vi "MGCC_StaEst_main.vi"() -> ()   [LabVIEW 2016]
panel:
  out "Boolean 7":bool
  out "Boolean 6":bool
  out "Boolean 5":bool
  out "Boolean 4":bool
  out "Boolean 3":bool
  out "Boolean 2":bool
  out "Boolean":bool
  out "Boolean":bool
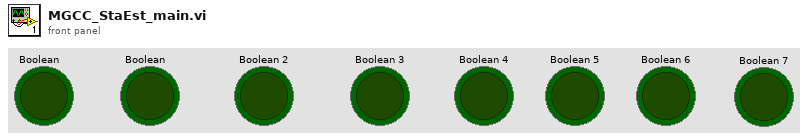
[diagram p1: front panel]
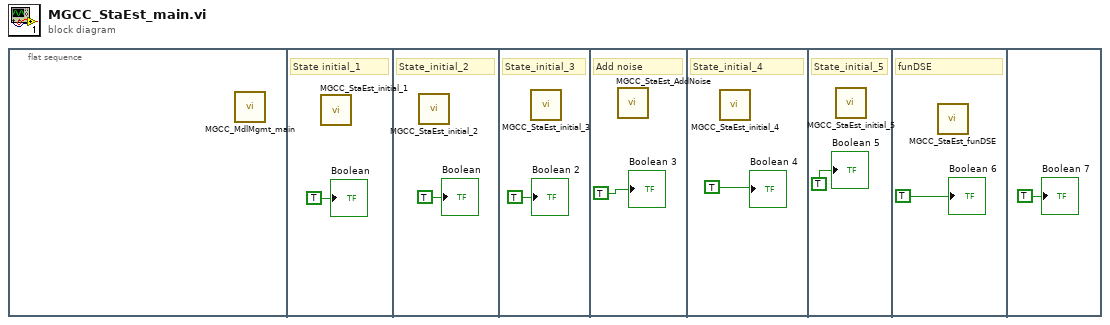
[diagram p0: block diagram]
diagram:
  n1 = flat-sequence {
    frame #0 {
      n2 = call "MGCC_MdlMgmt_main.vi"() -> ()  [unwired: 12 in]
    }
    frame #1 {
      # "State initial_1"
      n3 = call "MGCC_StaEst_initial_1.vi"() -> ()  [unwired: 6 in]
      "Boolean" <- TRUE ("Boolean")
    }
    frame #2 {
      # "State_initial_2"
      n4 = call "MGCC_StaEst_initial_2.vi"() -> ()  [unwired: 12 in]
      "Boolean" <- TRUE ("Boolean")
    }
    frame #3 {
      # "State_initial_3"
      n5 = call "MGCC_StaEst_initial_3.vi"() -> ()  [unwired: 12 in]
      "Boolean 2" <- TRUE ("Boolean 2")
    }
    frame #4 {
      # "Add noise"
      n6 = call "MGCC_StaEst_AddNoise.vi"() -> ()  [unwired: 12 in]
      "Boolean 3" <- TRUE ("Boolean 4")
    }
    frame #5 {
      # "State_initial_4"
      n7 = call "MGCC_StaEst_initial_4.vi"() -> ()  [unwired: 12 in]
      "Boolean 4" <- TRUE ("Boolean 5")
    }
    frame #6 {
      # "State_initial_5"
      n8 = call "MGCC_StaEst_initial_5.vi"() -> ()  [unwired: 12 in]
      "Boolean 5" <- TRUE ("Boolean 6")
    }
    frame #7 {
      # "funDSE"
      n9 = call "MGCC_StaEst_funDSE.vi"() -> ()  [unwired: 12 in]
      "Boolean 6" <- TRUE ("Boolean 7")
    }
    frame #8 {
      "Boolean 7" <- TRUE ("Boolean 7")
    }
  }
